vi "22-Host Sends Information to Equipment.vi"(8 "error in (no error)":errorcluster, 10 "TEXT":string, 11 "TID":u8) -> (0 "error out":errorcluster, 2 "Timeout?":bool, 3 "S10F4":T1)   [LabVIEW 2020, in "SECS Scenarios.lvlib" / "Scenarios Class.lvclass"]
uses:
  Scenarios Class.lvclass
  SECS Communication/S10 Message Class/S10F4.ctl
  22-Host Sends Information to Equipment.ctl
  SECS Communication/S10 Message Class/S10 Message Class.lvclass
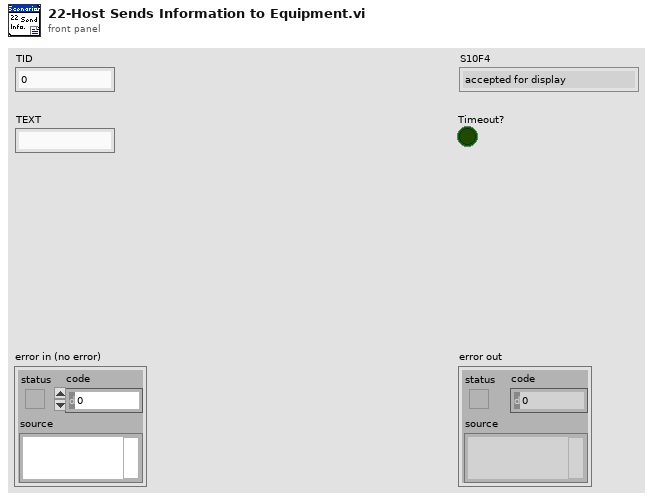
[diagram p1: front panel]
types:
  T1 = typedef "SECS Communication.lvlib/S10 Message Class.lvclass/S10F4.ctl" = enum8{"accepted for display", "message will not be displayed", "terminal not available"}
  T2 = typedef "SECS Scenarios.lvlib/Scenarios Class.lvclass/22-Host Sends Information to Equipment.ctl" = cluster{"TID":u8, "TEXT":string, "Reply Notifier":refnum<notifier>}
  T3 = typedef "SECS Scenarios.lvlib/Scenarios Class.lvclass/Broadcast Refnum.ctl" = cluster{"13-EnableDisable Alarm":refnum<user-event>, "15-Process Program Request":refnum<user-event>, "16-Process Program Send":refnum<user-event>, "17-Deleting a Process Program by Host":refnum<user-event>, "18-Host Requests Equipment Process Program Directory":refnum<user-event>, "19-Equipment Process Program Uploading":refnum<user-event>, "20[1]-Process Program Downloading":refnum<user-event>, "20[2]-Process Program Downloading":refnum<user-event>, "22-Host Sends Information to Equipment":refnum<user-event>, "26-Host Requests to Enter OFF-Line":refnum<user-event>, "27-Host Requests to Enter On-Line":refnum<user-event>, "28[1]-Remote Control[PP-SELECT]":refnum<user-event>, "28[2]-Remote Control[START]":refnum<user-event>, "28[3]-Remote Control[STOP]":refnum<user-event>, "28[4]-Remote Control[LOCAL]":refnum<user-event>, "28[5]-Remote Control[REMOTE]":refnum<user-event>, "28[6]-Remote Control[RCMD]":refnum<user-event>, "30-Host Requests Equipment to Set Time":refnum<user-event>, "31-Host Requests Time Value from Equipment":refnum<user-event>, "32[1]-Trace Data Collection":refnum<user-event>, "32[2]-Trace Data Collection":refnum<user-event>}
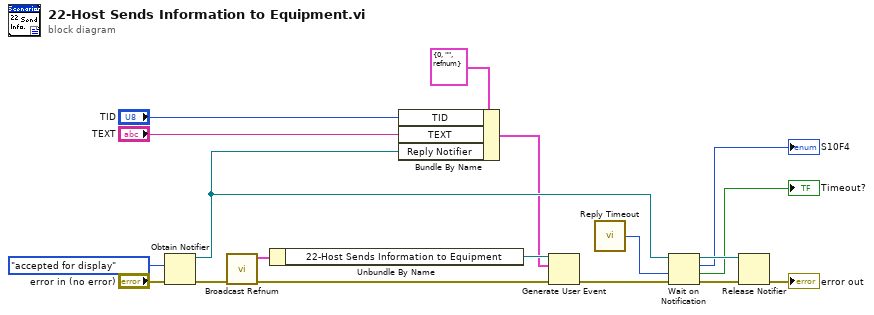
[diagram p0: block diagram]
diagram:
  n1 = Obtain Notifier(notification data type=S10F4."accepted for display" ("S10F4"), error in (no error)="error in (no error)") -> (notifier out=w7:refnum<notifier>, error out=w17:errorcluster)  [unwired: 2 in, 1 out]
  n2 = call "Broadcast Refnum.vi"("error in"=w17) -> ("error out"=w16:errorcluster, "Broadcast Refnum"=w18:T3)  [unwired: 9 in]
  n3 = Unbundle By Name(w18) -> ("22-Host Sends Information to Equipment"=w15:refnum<user-event>)
  n4 = Bundle By Name(cluster=T2 {"TID"=0, "TEXT"="", "Reply Notifier"=refnum} ("22-Host Sends Information to Equipment"), "TID"="TID", "TEXT"="TEXT", "Reply Notifier"=w7) -> (w2:T2)
  n5 = Generate User Event(user event=w15, event data cluster=w2, error in=w16) -> (error out=w14:errorcluster)  [unwired: 1 in, 1 out]
  n6 = call "Reply Timeout.vi"() -> ("Reply Timeout"=w13:i32)
  n7 = Wait on Notification(notifier=w7, timeout in ms (-1)=w13, error in (no error)=w14) -> (notifier out=w12:refnum<notifier>, notification=→"S10F4":T1, timed out?=→"Timeout?":bool, error out=w11:errorcluster)  [unwired: 1 in]
  n8 = Release Notifier(notifier=w12, error in (no error)=w11) -> (error out=→"error out":errorcluster)  [unwired: 1 in, 2 out]
